vi "Corr_stats_labels.vi"(2 "Inst 2 Units":T1={"Colour"=0, "Inst type"=enum."Pitot-static tube", "Inst name"="Manometer voltage", "Symbol"="U", "Code name"="", "Extra Info"="U", "Inst Array"=enum."PWA", "Extra Titles"=[], "Extra Values"=[], "U"=0.0, "u^2"=0.0, "u^3"=0.0, "u^4"=0.0, "Skew_u"=0.0, "Kurt_u"=0.0, "Sd Error in Mean"=0.0, "% u'/U"=0.0, "X"=0.0, "Y"=0.0, "Z"=0.0, "Timescale integral to 25%"=0.0, "Sd Error in Variance"=0.0, "Calib File"=path "", "Calib Constants"=[], "Output Position"=FALSE, "Full Stats"=FALSE, "Av Sampling Rate"=0.0, "Av No of Samples"=0.0, "Total Meas Time (s)"=0.0, "ADAM Ch Name"=""} {"Sd Error in Variance" format="%.2f"; "Skew_u" format="%.2f"; "% u'/U" format="%.2f"; "Sd Error in Mean" format="%.2f"; "Kurt_u" format="%.2f"; "u^4" format="%.2f"; "u^3" format="%.2f"; "U" format="%.2f"; "u^2" format="%.2f"}, 3 "Inst 1 Units":T1={"Colour"=0, "Inst type"=enum."Pitot-static tube", "Inst name"="Manometer voltage", "Symbol"="U", "Code name"="", "Extra Info"="U", "Inst Array"=enum."PWA", "Extra Titles"=[], "Extra Values"=[], "U"=0.0, "u^2"=0.0, "u^3"=0.0, "u^4"=0.0, "Skew_u"=0.0, "Kurt_u"=0.0, "Sd Error in Mean"=0.0, "% u'/U"=0.0, "X"=0.0, "Y"=0.0, "Z"=0.0, "Timescale integral to 25%"=0.0, "Sd Error in Variance"=0.0, "Calib File"=path "", "Calib Constants"=[], "Output Position"=FALSE, "Full Stats"=FALSE, "Av Sampling Rate"=0.0, "Av No of Samples"=0.0, "Total Meas Time (s)"=0.0, "ADAM Ch Name"=""} {"Sd Error in Variance" format="%.2f"; "Skew_u" format="%.2f"; "% u'/U" format="%.2f"; "Sd Error in Mean" format="%.2f"; "Kurt_u" format="%.2f"; "u^4" format="%.2f"; "u^3" format="%.2f"; "U" format="%.2f"; "u^2" format="%.2f"}) -> (0 "Output":string[](array[string]))   [LabVIEW 2012]
uses:
  Controls/Analysis_info_cluster.ctl
  Controls/Inst_type.ctl
  Controls/Instrument_Array.ctl
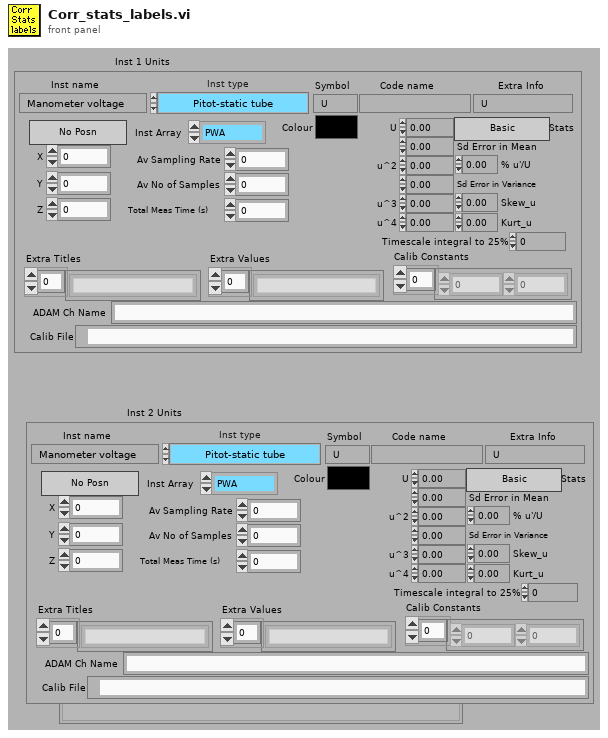
[diagram p1: front panel]
types:
  T1 = typedef "Analysis_info_cluster.ctl" = cluster{"Colour":u32, "Inst type":T2, "Inst name":string, "Symbol":string, "Code name":string, "Extra Info":string, "Inst Array":T3, "Extra Titles":string[], "Extra Values":string[], "U":dbl, "u^2":dbl, "u^3":dbl, "u^4":dbl, "Skew_u":dbl, "Kurt_u":dbl, "Sd Error in Mean":dbl, "% u'/U":dbl, "X":dbl, "Y":dbl, "Z":dbl, "Timescale integral to 25%":dbl, "Sd Error in Variance":dbl, "Calib File":path, "Calib Constants":dbl[], "Output Position":bool, "Full Stats":bool, "Av Sampling Rate":dbl, "Av No of Samples":dbl, "Total Meas Time (s)":dbl, "ADAM Ch Name":string}
  T2 = typedef "Inst_type.ctl" = enum16{"Propeller anemometer", "Raw voltage", "Pressure Transducer", "Pitot-static tube", "Preston tube", "Hot wire", "Cross wire 1", "Cross wire 2", "Generic Linear", "Generic Polynomial", "Generic BackPoly", "Fast FID", "Thermocouple", "Cold wire", "Pulsed Wire", "LDA Vel", "LDA Tran time", "LDA Arr time"}
  T3 = typedef "Instrument_Array.ctl" = enum16{"PWA", "LDA", "Analogue"}
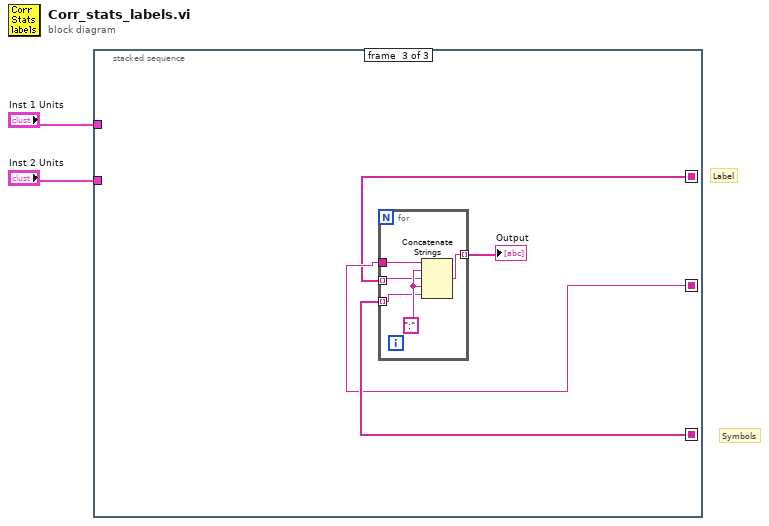
[diagram p0: block diagram]
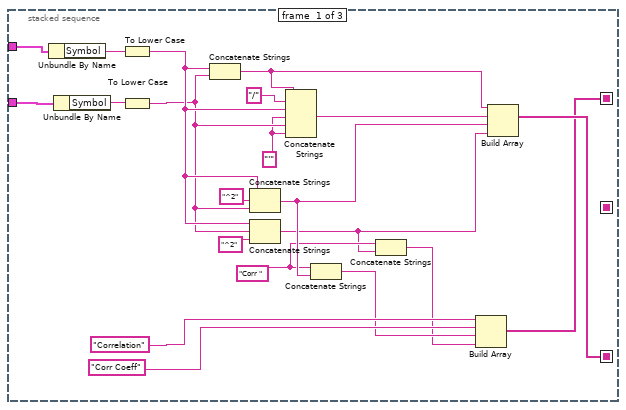
[diagram p2: hidden frame]
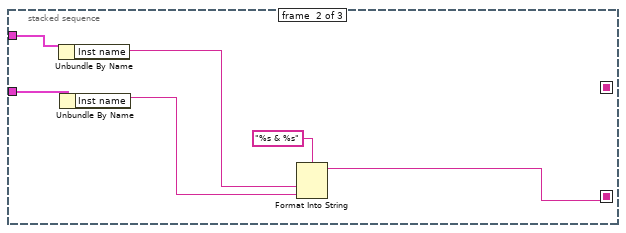
[diagram p3: hidden frame]
diagram:
  # "Label"
  # "Symbols"
  n1 = stacked-sequence {
    seq-local: [w15 _ _] -> [_ _ w33]
    seq-local: [w14 _ _] -> [_ _ w30]
    seq-local: [_ w24 _] -> [_ _ w31]
    tunnel: "Inst 2 Units" -> [w19 w28 _]
    tunnel: "Inst 1 Units" -> [w16 w29 _]
    frame #0 {
      w5 = "Corr "
      w9 = "'"
      n2 = Unbundle By Name(w16) -> ("Symbol"=w18:string)
      n3 = Unbundle By Name(w19) -> ("Symbol"=w17:string)
      n4 = To Lower Case(string=w18) -> (all lower case string=w23:string)
      n5 = To Lower Case(string=w17) -> (all lower case string=w22:string)
      n6 = Concatenate Strings(w23, w22) -> (w11:string)
      n7 = Concatenate Strings(w23, "^2", w22) -> (w7:string)
      n8 = Concatenate Strings(w23, w22, "^2") -> (w4:string)
      n9 = Concatenate Strings(w11, "/", w23, w9, w22, w9) -> (w8:string)
      n10 = Concatenate Strings(w5, w7) -> (w6:string)
      n11 = Concatenate Strings(w5, w4) -> (w3:string)
      n12 = Build Array("Correlation", "Corr Coeff", w6, w3) -> (w14:string[])
      n13 = Build Array(w11, w8, w7, w4) -> (w15:string[])
    }
    frame #1 {
      n14 = Unbundle By Name(w29) -> ("Inst name"=w26:string)
      n15 = Unbundle By Name(w28) -> ("Inst name"=w25:string)
      n16 = Format Into String(format string="%s & %s" ("Format String"), w26, w25) -> (resulting string=w24:string)  [unwired: 2 in, 1 out]
    }
    frame #2 {
      n17 = for {
        tunnel: [w38] -> w32 mode=indexing
        tunnel: w31 -> [w37]
        tunnel: w30 -> [w35] mode=indexing
        tunnel: w33 -> [w34] mode=indexing
        w36 = ":" ("Substring")
        n18 = Concatenate Strings(w37, w36, w35, w36, w34) -> (w38:string)
      }
      "Output" <- w32
    }
  }
